vi "Filter and Log Error.vi"(8 "error In":errorcluster, 11 "Full Name":string="CIF Plugin Loader") -> ()   [LabVIEW 2021, in "CIFPluginLoaderClientWrapper.lvlib"]
uses:
  CIFPluginLoaderClientWrapper.lvlib
  CIFUtilities/CIFLogs/CIFLogs.lvlib
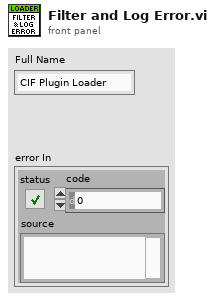
[diagram p1: front panel]
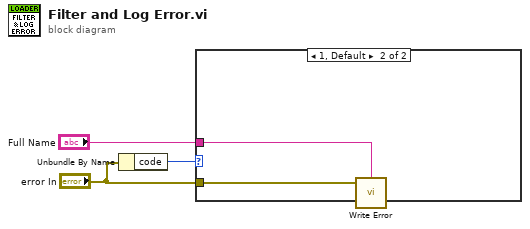
[diagram p0: block diagram]
diagram:
  n1 = Unbundle By Name("error In") -> ("code"=w3:i32)
  n2 = case shown="1, Default" w3 {
    tunnel: "error In" -> [_ w5]
    tunnel: "Full Name" -> [_ w4]
    frame -1001, -2, 0 {
      # "-1001 is cancelled by client.  Not an error.\n-2 (Invalid Argument) can be caused by race condition on client timeout."
    }
    frame 1, Default {
      n3 = call "Write Error.vi"("error in (no error)"=w5, "Plugin Name"=w4) -> ()  [unwired: 2 in, 1 out]
    }
  }
